vi "NI 5413 initialise.vi"(5 "Channel":string="0", 6 "Source (Onboard Clock)":T1="OnboardClock", 7 "Standard Waveform":u16(ring) items=["Sine", "Square", "Triangle", "Ramp Up", "Ramp Down", "DC", "Noise"], 8 "error in (no error)":errorcluster, 9 "Amplitude":dbl=2.0 format="%0_3g", 10 "Frequency":dbl=1000000.0 format="%.2p", 11 "FGEN Resource Name":refnum<k15>) -> (0 "error out":errorcluster, 3 "Instrument Handle Out":refnum<k15>)   [LabVIEW 2020]
doc: "This example shows how to use Standard Function mode. This is a basic example that shows the smallest amount of code necessary to generate a standard waveform."
uses:
  <instrlib>/niFgen/niFgen.llb/niFgen_ctl Sample Clock Source Values (Ring).ctl
  <instrlib>/niFgen/niFgen.llb/niFgen Output Mode.ctl
panel:
  # "Overview: Demonstrates how to configure an NI Signal Source to generate a basic standard function.\nSoftware Requirements: NI-FGEN\nHardware Requirements: PXI-5401, PCI-5401, PXI-5402, PCI-5402, PXI-5406, PCI-5406, PXI-5411, PCI-5411, AT-5411, PXI-5412, PCI-5412, PXIe-5413, PXI-5421, PCI-5421, PXI-5422, PXIe-5423, PXI-5431, PCI-5431, PXIe-5433, PXI-5441, NI PXIe-5442, NI PXIe-5450, or NI PXIe-5451 \nInstructions:\n1. Select the FGEN Resource Name as configured in the Measurement & Automation Explorer.\n2. Select the Standard Waveform to be generated.\n3. Specify the desired Frequency for the waveform.\n4. Select to Amplitude of the waveform.\n5. Run the VI.\n6. Click Stop to stop the VI."
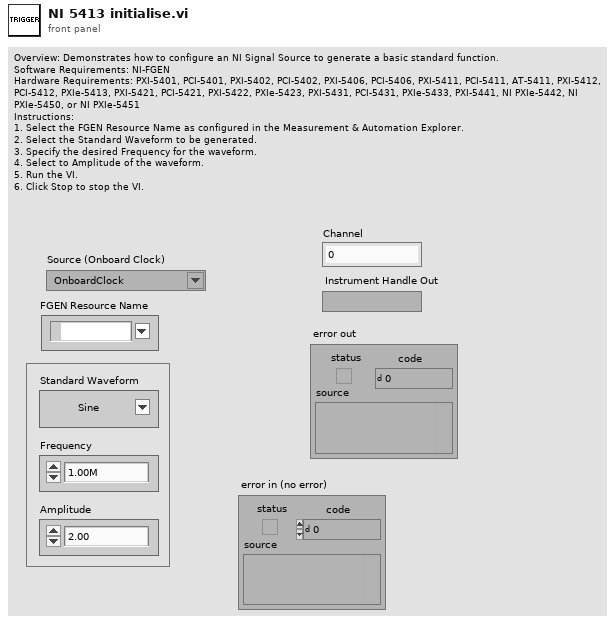
[diagram p1: front panel]
types:
  T1 = typedef "niFgen_ctl Sample Clock Source Values (Ring).ctl" = string
  T2 = typedef "niFgen Output Mode.ctl" = u32
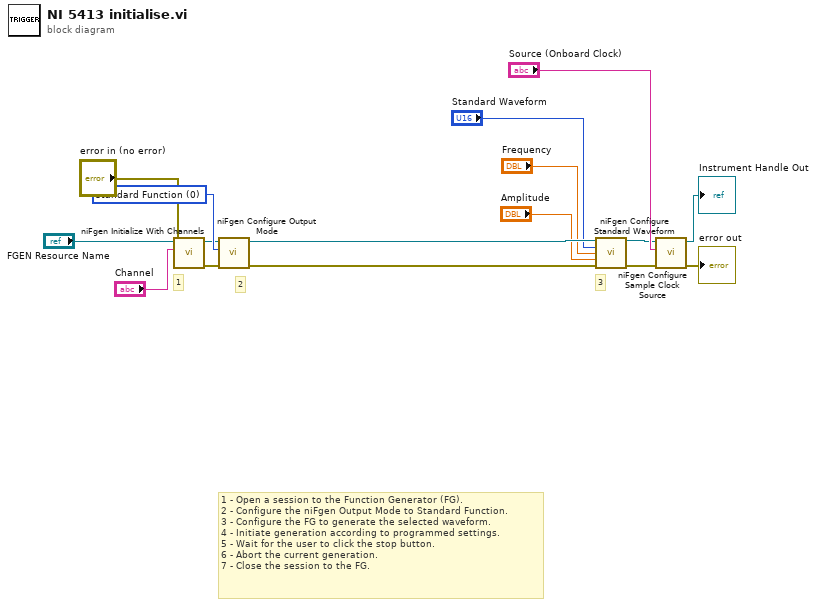
[diagram p0: block diagram]
diagram:
  w16 = T2 0 items=["Standard Function", "Frequency List", "Arbitrary Waveform", "Arbitrary Sequence", "Script"] ("output mode")
  # "3"
  # "2"
  # "1"
  # "1 - Open a session to the Function Generator (FG).\n2 - Configure the niFgen Output Mode to Standard Function.\n3 - Configure the FG to generate the selected waveform.\n4 - Initiate generation according to programmed settings.\n5 - Wait for the user to click the stop button.\n6 - Abort the current generation.\n7 - Close the session to the FG."
  n1 = call <instrlib>:"niFgen Initialize With Channels.vi"("error in (no error)"="error in (no error)", "Channel Name"="Channel", "Resource Name"="FGEN Resource Name") -> ("error out"=w8:errorcluster, "Instrument Handle Out"=w9:refnum<k15>)  [unwired: 7 in]
  n2 = call <instrlib>:"niFgen Configure Output Mode.vi"("error in (no error)"=w8, "Output Mode (default: 0=Standard Function)"=w16, "Instrument Handle"=w9) -> ("error out"=w14:errorcluster, "Instrument Handle Out"=w15:refnum<k15>)  [unwired: 6 in]
  n3 = call <instrlib>:"niFgen Configure Standard Waveform.vi"("Instrument Handle"=w15, "Waveform"="Standard Waveform", "Frequency"="Frequency", "Amplitude"="Amplitude", "error in (no error)"=w14) -> ("Instrument Handle Out"=w4:refnum<k15>, "error out"=w5:errorcluster)  [unwired: 9 in]
  n4 = call <instrlib>:"niFgen Configure Sample Clock Source.vi"("error in (no error)"=w5, "Source (Onboard Clock)"="Source (Onboard Clock)", "Instrument Handle"=w4) -> ("error out"=→"error out":errorcluster, "Instrument Handle Out"=→"Instrument Handle Out":refnum<k15>)  [unwired: 7 in]
